vi "Get Impulse Data.vi"(10 "Channel":i32, 11 "Reference in":T1) -> (1 "Impulses out":dbl[][](array[numeric]), 3 "Reference out":T1)   [LabVIEW 2016, in "Impulse Data.lvclass"]
uses:
  Impulse Data.lvclass
  Instance handle.ctl
  Impulse Data.lvclass/Impulse Data.ctl
  Abstract Data Manipulator/Abstract Data Manipulator.lvclass
panel:
  out "error out":errorcluster
  in  "error in (no error)":errorcluster
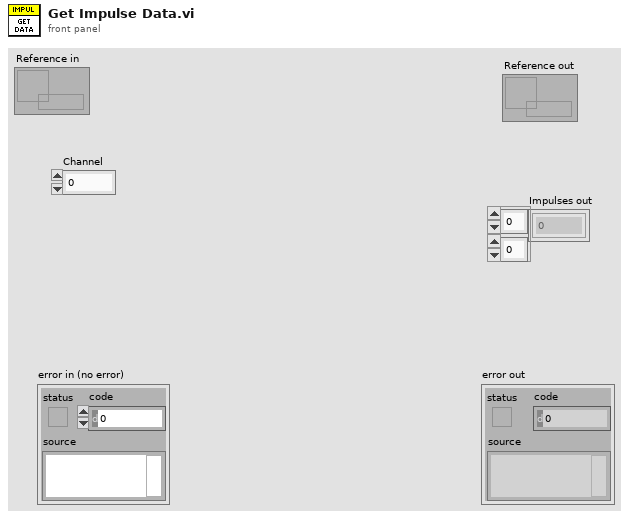
[diagram p1: front panel]
types:
  T1 = typedef "Impulse Data.lvclass/Instance handle.ctl" = refnum<data-value>
  T2 = typedef "TD_Impulse Planes.ctl" = enum16{"Other", "Yaw", "Pitch", "Roll", "LARP", "RALP"}
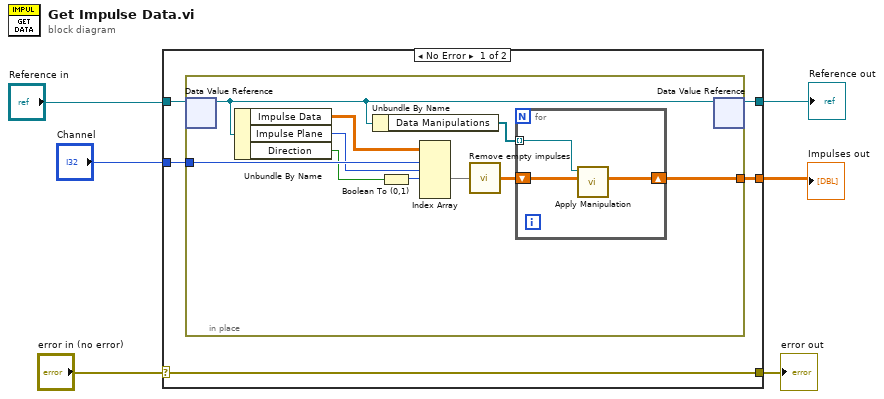
[diagram p0: block diagram]
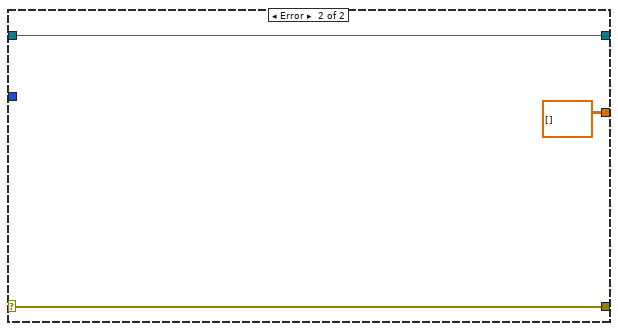
[diagram p2: hidden frame]
diagram:
  n1 = case shown="No Error" "error in (no error)" {
    selector: "error in (no error)" -> [w11 w27]
    tunnel: [w11 w27] -> w5
    tunnel: [w9 w26] -> w4
    tunnel: "Reference in" -> [w10 w26]
    tunnel: "Channel" -> [w8 _]
    tunnel: [w7 dbl[][] [] ("Impulse Data")] -> w1
    frame No Error {
      n2 = in-place {
        in-place-border: w8 -> [w20]
        in-place-border: [w17] -> w7
        n3 = in-place-dvr #1(w10) -> (w19:refnum<class "Impulse Data.lvclass">)  [unwired: 1 out]
        n4 = Unbundle By Name(w19) -> ("Impulse Data"=w21:dbl[][][][][], "Impulse Plane"=w14:T2, "Direction"=w16:bool)
        n5 = Unbundle By Name(w19) -> ("Data Manipulations"=w18:refnum<class "Abstract Data Manipulator.lvclass">[])
        n6 = Boolean To (0,1)(Boolean=w16) -> (0, 1=w15:i16)
        n7 = Index Array(array=w21, index (dim 0)=w20, index (dim 1)=w14, index (dim 2)=w15) -> (element=w13:dbl[][])  [unwired: 2 in]
        n8 = call "Remove empty impulses.vi"("Data out"=w13) -> ("Data out 2"=w12:dbl[][])
        n9 = for {
          tunnel: w18 -> [w24] mode=indexing
          shift-right: [w22] -> w17
          shift-left: w12 -> [w23]
          n10 = call-dynamic "Apply Manipulation.vi"("Data in"=w23, "Abstract Data Manipulator in"=w24) -> ("Data out"=w22:dbl[][])  [unwired: 7 in, 2 out]
        }
        n11 = in-place-dvr #1(w19) -> (w9:T1)  [unwired: 1 out]
      }
    }
    frame Error {
    }
  }
  "error out" <- w5
  "Reference out" <- w4
  "Impulses out" <- w1
